vi "VI Tree.vi"   [LabVIEW 2010, in "Agilent 4194.lvlib"]
doc: "This is the LabVIEW Instrument Driver for the Hewlett-Packard 4194A Impedance/Gain-Phase Analyzer. The VI Tree displays all the user-callable VIs of the instrument driver in an organized table."
uses:
  <instrlib>/Agilent 4194/Agilent 4194.lvlib
panel:
  # "© 2005 National Instruments.  ALL RIGHTS RESERVED."
  # "SEE DIAGRAM\nFOR VI TREE."
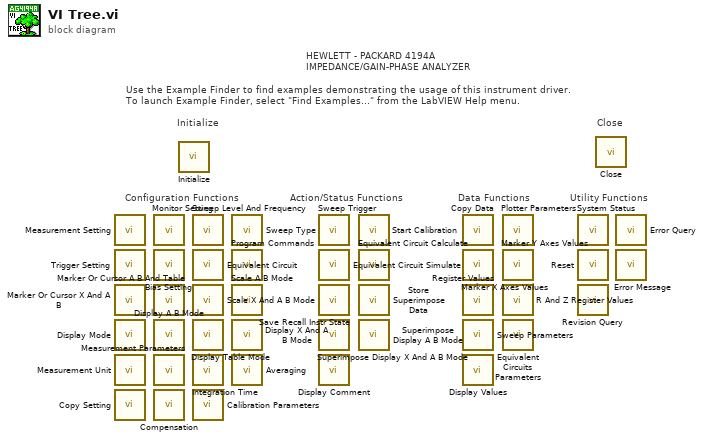
[diagram p0: block diagram]
diagram:
  # "Utility Functions"
  # "Data Functions"
  # "Action/Status Functions"
  # "Configuration Functions"
  # "Close"
  # "Use the Example Finder to find examples demonstrating the usage of this instrument driver.\nTo launch Example Finder, select \"Find Examples...\" from the LabVIEW Help menu."
  # "Initialize"
  # "HEWLETT - PACKARD 4194A\nIMPEDANCE/GAIN-PHASE ANALYZER"
  n1 = call <instrlib>:"Measurement Setting.vi"() -> ()  [unwired: 10 in, 2 out]
  n2 = call <instrlib>:"Trigger Setting.vi"() -> ()  [unwired: 10 in, 2 out]
  n3 = call <instrlib>:"Marker Or Cursor X And A B.vi"() -> ()  [unwired: 18 in, 2 out]
  n4 = call <instrlib>:"Display Mode.vi"() -> ()  [unwired: 10 in, 2 out]
  n5 = call <instrlib>:"Measurement Unit.vi"() -> ()  [unwired: 10 in, 2 out]
  n6 = call <instrlib>:"Copy Setting.vi"() -> ()  [unwired: 14 in, 2 out]
  n7 = call <instrlib>:"Monitor Setting.vi"() -> ()  [unwired: 10 in, 2 out]
  n8 = call <instrlib>:"Bias Setting.vi"() -> ()  [unwired: 10 in, 2 out]
  n9 = call <instrlib>:"Marker Or Cursor A B And Table.vi"() -> ()  [unwired: 10 in, 2 out]
  n10 = call <instrlib>:"Display A B Mode.vi"() -> ()  [unwired: 14 in, 2 out]
  n11 = call <instrlib>:"Measurement Parameters.vi"() -> ()  [unwired: 10 in, 2 out]
  n12 = call <instrlib>:"Compensation.vi"() -> ()  [unwired: 10 in, 2 out]
  n13 = call <instrlib>:"Initialize.vi"() -> ()  [unwired: 10 in, 2 out]
  n14 = call <instrlib>:"Sweep Level And Frequency.vi"() -> ()  [unwired: 14 in, 2 out]
  n15 = call <instrlib>:"Equivalent Circuit.vi"() -> ()  [unwired: 14 in, 2 out]
  n16 = call <instrlib>:"Scale X And A B Mode.vi"() -> ()  [unwired: 14 in, 2 out]
  n17 = call <instrlib>:"Display Table Mode.vi"() -> ()  [unwired: 10 in, 2 out]
  n18 = call <instrlib>:"Integration Time.vi"() -> ()  [unwired: 10 in, 2 out]
  n19 = call <instrlib>:"Calibration Parameters.vi"() -> ()  [unwired: 10 in, 2 out]
  n20 = call <instrlib>:"Sweep Type.vi"() -> ()  [unwired: 10 in, 2 out]
  n21 = call <instrlib>:"Program Commands.vi"() -> ()  [unwired: 10 in, 2 out]
  n22 = call <instrlib>:"Scale A B Mode.vi"() -> ()  [unwired: 14 in, 2 out]
  n23 = call <instrlib>:"Display X And A B Mode.vi"() -> ()  [unwired: 14 in, 2 out]
  n24 = call <instrlib>:"Averaging.vi"() -> ()  [unwired: 10 in, 2 out]
  n25 = call <instrlib>:"Sweep Trigger.vi"() -> ()  [unwired: 10 in, 2 out]
  n26 = call <instrlib>:"Equivalent Circuit Simulate.vi"() -> ()  [unwired: 10 in, 2 out]
  n27 = call <instrlib>:"Save Recall Instr State.vi"() -> ()  [unwired: 10 in, 2 out]
  n28 = call <instrlib>:"Superimpose Display X And A B Mode.vi"() -> ()  [unwired: 10 in, 2 out]
  n29 = call <instrlib>:"Display Comment.vi"() -> ()  [unwired: 10 in, 2 out]
  n30 = call <instrlib>:"Start Calibration.vi"() -> ()  [unwired: 10 in, 2 out]
  n31 = call <instrlib>:"Equivalent Circuit Calculate.vi"() -> ()  [unwired: 10 in, 2 out]
  n32 = call <instrlib>:"Store Superimpose Data.vi"() -> ()  [unwired: 10 in, 2 out]
  n33 = call <instrlib>:"Superimpose Display A B Mode.vi"() -> ()  [unwired: 10 in, 2 out]
  n34 = call <instrlib>:"Copy Data.vi"() -> ()  [unwired: 10 in, 2 out]
  n35 = call <instrlib>:"Marker X Axes Values.vi"() -> ()  [unwired: 7 in, 5 out]
  n36 = call <instrlib>:"Register Values.vi"() -> ()  [unwired: 6 in, 6 out]
  n37 = call <instrlib>:"Sweep Parameters.vi"() -> ()  [unwired: 4 in, 8 out]
  n38 = call <instrlib>:"Display Values.vi"() -> ()  [unwired: 4 in, 8 out]
  n39 = call <instrlib>:"Plotter Parameters.vi"() -> ()  [unwired: 10 in, 2 out]
  n40 = call <instrlib>:"Marker Y Axes Values.vi"() -> ()  [unwired: 8 in, 12 out]
  n41 = call <instrlib>:"R And Z Register Values.vi"() -> ()  [unwired: 8 in, 4 out]
  n42 = call <instrlib>:"Equivalent Circuits Parameters.vi"() -> ()  [unwired: 6 in, 6 out]
  n43 = call <instrlib>:"System Status.vi"() -> ()  [unwired: 8 in, 4 out]
  n44 = call <instrlib>:"Reset.vi"() -> ()  [unwired: 10 in, 2 out]
  n45 = call <instrlib>:"Revision Query.vi"() -> ()  [unwired: 8 in, 4 out]
  n46 = call <instrlib>:"Close.vi"() -> ()  [unwired: 11 in, 1 out]
  n47 = call <instrlib>:"Error Query.vi"() -> ()  [unwired: 8 in, 4 out]
  n48 = call <instrlib>:"Error Message.vi"() -> ()  [unwired: 7 in, 5 out]
